vi "VentState.vi"(8 "error in (no error)":errorcluster, 10 "Cluster in":T2, 11 "Enum in":T1) -> (0 "error out":errorcluster, 2 "Cluster out":T2, 3 "Enum out":T1)   [LabVIEW 2018]
uses:
  Type_Def Actuator Controls.ctl
  Type_Def_ControlState.ctl
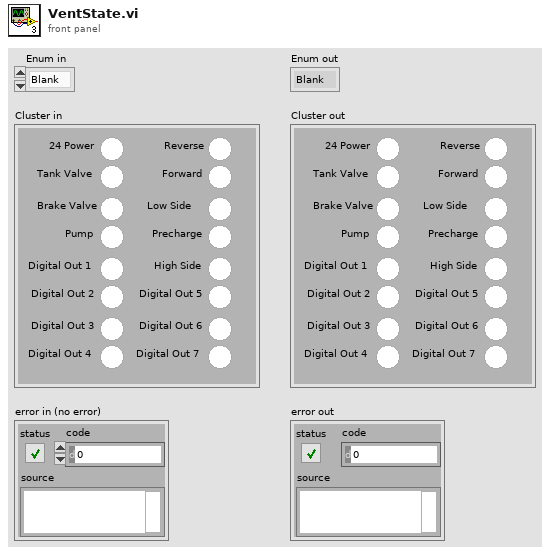
[diagram p1: front panel]
types:
  T1 = typedef "Type_Def_ControlState.ctl" = enum16{"Blank", "Systems Check", "Idle", "Ready", "Pushing", "CrawlingPrecharge", "Braking", "Fault", "Boot Up", "Unpowered", "Crawling", "Shutdown", "Service Push", "Service Wait", "Vent", "Precharge", "Cooldown"}
  T2 = typedef "Type_Def Actuator Controls.ctl" = cluster{"Reverse ":bool, "Forward":bool, "Low Side":bool, "Precharge":bool, "High Side":bool, "Digital Out 5":bool, "Digital Out 6":bool, "Digital Out 7 ":bool, "24 Power":bool, "Tank Valve ":bool, "Brake Valve":bool, "Pump":bool, "Digital Out 1 ":bool, "Digital Out 2":bool, "Digital Out 3":bool, "Digital Out 4 ":bool}
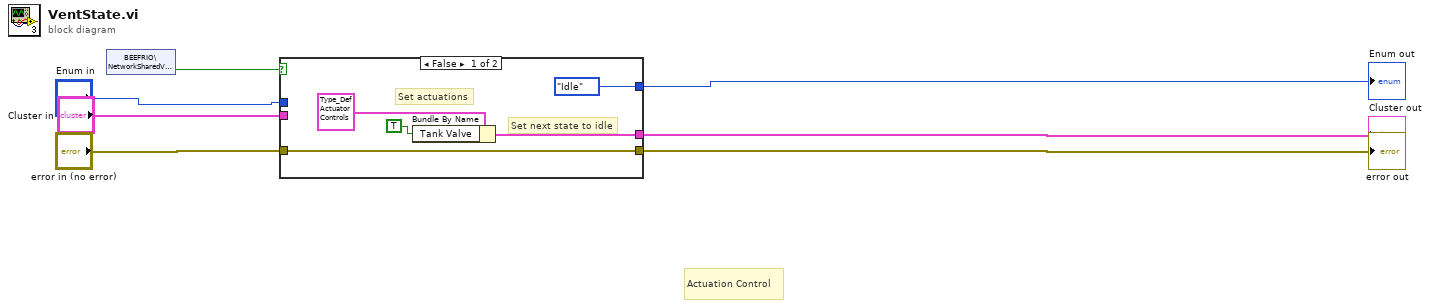
[diagram p0: block diagram]
diagram:
  # "Actuation Control"
  n1 = shared-variable "BEEFRIO\\NetworkSharedVariable.lvlib\\Vent"() -> (w7:bool)  [unwired: 1 in, 1 out]
  n2 = case shown="False" w7 {
    tunnel: "Enum in" -> [_ w15]
    tunnel: [Type_Def_ControlState."Idle" w15] -> w2
    tunnel: "Cluster in" -> [_ w14]
    tunnel: [w10 w14] -> w4
    tunnel: [w9 w13] -> w5
    tunnel: "error in (no error)" -> [w9 w13]
    frame False {
      # "Set next state to idle"
      # "Set actuations"
      n3 = Bundle By Name(cluster=T2 {"Reverse "=FALSE, "Forward"=FALSE, "Low Side"=FALSE, "Precharge"=FALSE, "High Side"=FALSE, "Digital Out 5"=FALSE, "Digital Out 6"=FALSE, "Digital Out 7 "=FALSE, "24 Power"=FALSE, "Tank Valve "=FALSE, "Brake Valve"=FALSE, "Pump"=FALSE, "Digital Out 1 "=FALSE, "Digital Out 2"=FALSE, "Digital Out 3"=FALSE, "Digital Out 4 "=FALSE} ("Cluster in"), "Tank Valve"=TRUE ("Digital Out 5")) -> (w10:T2)
    }
    frame True {
      # "Pass next vent through agian"
    }
  }
  "error out" <- w5
  "Cluster out" <- w4
  "Enum out" <- w2
